vi "polhemus_only.vi"() -> ()   [LabVIEW 2017]
uses:
  <instrlib>/PDI/pdi.llb/PDI motion data.ctl
  <instrlib>/PDI/pdi.llb/PDI BINHDR.ctl
  <instrlib>/PDI/pdi.llb/PDI 6vec.ctl
  <instrlib>/PDI/pdi.llb/PDI counter.ctl
  <instrlib>/PDI/pdi.llb/PDI flag.ctl
  <instrlib>/PDI/pdi.llb/PDI DirCos cluster.ctl
  <instrlib>/PDI/pdi.llb/PDI quaternion.ctl
  <vilib>/Utility/file.llb/Write Delimited Spreadsheet (DBL).vi
panel:
  in  "file name":string
  in  "Path":path
  out "Continuing":bool
  in  "Stop Collect":bool
  out "motion data":T1 {"QT array"."Numeric 4" format="%_6g"; "QT array"."Numeric 3" format="%_6g"; "QT array"."Numeric 2" format="%_6g"; "QT array"."Numeric" format="%_6f"; "DC array"."Z"."z" format="%1_6f"; "DC array"."Z"."Y" format="%1_6f"; "DC array"."Z"."X" format="%1_6f"; "DC array"."Y"."z" format="%1_6f"; "DC array"."Y"."Y" format="%1_6f"; "DC array"."Y"."X" format="%1_6f"; "DC array"."X"."Z" format="%1_6f"; "DC array"."X"."Y" format="%1_6f"; "DC array"."X"."X" format="%1_6f"; "DL array" min=0 max=1 format="%.0g"; "ST array" min=0 max=1 format="%.0g"; "ES array" min=0 max=1 format="%.0g"; "TS array" format="%#.0g"; "FC array" format="%#.0g"; "XYZAER array"."R" format="%1_6f"; "XYZAER array"."E" format="%1_6f"; "XYZAER array"."A" format="%1_6f"; "XYZAER array"."Z" format="%1_6f"; "XYZAER array"."Y" format="%1_6f"; "XYZAER array"."X" format="%1_6f"; "BINHDR array"."Length" format="%04x"; "BINHDR array"."Reserved" format="%02x"; "BINHDR array"."Err" format="%02x"; "BINHDR array"."Cmd" format="%02x"; "BINHDR array"."Station" format="%02x"; "BINHDR array"."Preamble" format="%04x"}
  in  "Start Collect":bool
  in  "stop":bool
  out "error out":errorcluster {"code" format="%.0x"}
  out "Connected":bool
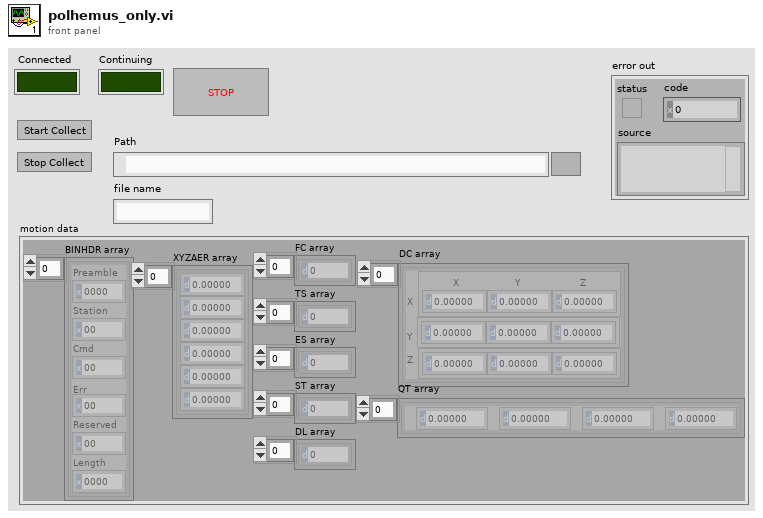
[diagram p1: front panel]
types:
  T1 = typedef "PDI motion data.ctl" = cluster{"BINHDR array":T2[], "XYZAER array":T3[], "FC array":T4[], "TS array":T4[], "ES array":T5[], "ST array":T5[], "DL array":T5[], "DC array":T6[], "QT array":T7[]}
  T2 = typedef "PDI BINHDR.ctl" = cluster{"Preamble":u16, "Station":u8, "Cmd":u8, "Err":u8, "Reserved":u8, "Length":u16}
  T3 = typedef "PDI 6vec.ctl" = cluster{"X":sgl, "Y":sgl, "Z":sgl, "A":sgl, "E":sgl, "R":sgl}
  T4 = typedef "PDI counter.ctl" = u32
  T5 = typedef "PDI flag.ctl" = i32
  T6 = typedef "PDI DirCos cluster.ctl" = cluster{"X":cluster{"X":sgl, "Y":sgl, "Z":sgl}, "Y":cluster{"X":sgl, "Y":sgl, "z":sgl}, "Z":cluster{"X":sgl, "Y":sgl, "z":sgl}}
  T7 = typedef "PDI quaternion.ctl" = cluster{"Numeric":sgl, "Numeric 2":sgl, "Numeric 3":sgl, "Numeric 4":sgl}
  T8 = enum16{"open", "open or create", "create or replace", "create", "open (read-only)"}
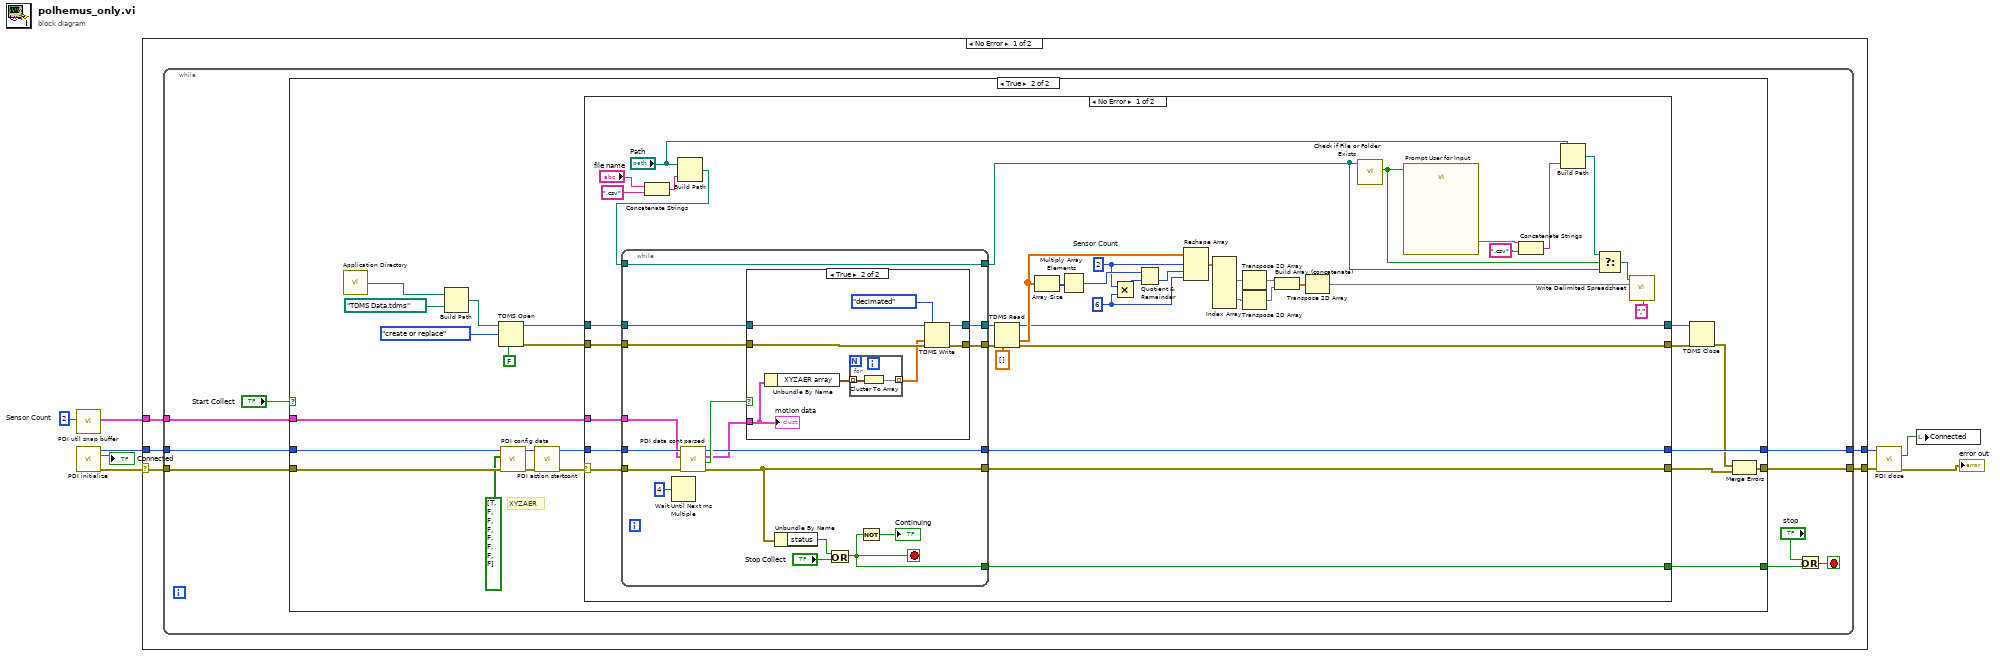
[diagram p0: block diagram]
diagram:
  w6 = 2  # Sensor Count
  n1 = call <instrlib>:"PDI util snap buffer.vi"("Sensor Count"=w6) -> ("snap buffer"=w7:T1)  [unwired: 8 in, 2 out]
  n2 = call <instrlib>:"PDI initialize.vi"() -> ("error out"=w4:errorcluster, "Connected"=→"Connected":bool, "pDev"=w8:u32)  [unwired: 5 in]
  n3 = case shown="No Error" w4 {
    selector: w4 -> [w11 w121]
    tunnel: [w14 w121] -> w3
    tunnel: [w13 w122] -> w5
    tunnel: w8 -> [w10 w122]
    tunnel: w7 -> [w12 _]
    frame No Error {
      n4 = while {
        tunnel: [w21] -> w14
        tunnel: [w20] -> w13
        tunnel: w12 -> [w19]
        tunnel: w11 -> [w18]
        tunnel: w10 -> [w17]
        stop <- w16 stop-if-true
        n5 = case shown="True" "Start Collect" {
          tunnel: [w24 w38] -> w21
          tunnel: [w25 w47] -> w20
          tunnel: w19 -> [_ w46]
          tunnel: w18 -> [w24 w32]
          tunnel: w17 -> [w25 w30]
          tunnel: [_ w27] -> w15
          frame False {
          }
          frame True {
            # "XYZAER"
            n6 = call <vilib>:"Application Directory.vi"() -> ("Application Directory"=w26:path)
            n7 = Build Path(base path=w26, name or relative path=path "TDMS Data.tdms" ("file path")) -> (appended path=w41:path)
            n8 = TDMS Open(6:FALSE ("disable buffering? (T)"), 10:T8."create or replace" ("operation"), 11:w41) -> (0:w44:errorcluster, 3:w45:refnum<k34>)  [unwired: 4 in]
            n9 = call <instrlib>:"PDI config data.vi"("error in (no error)"=w32, "Frame Data Select\nXYZAER    FC           TS           ES          ST           DL          DC          QT"=bool[] [TRUE, FALSE, FALSE, FALSE, FALSE, FALSE, FALSE, FALSE] ("Frame Data Select\nXYZAER    FC           TS           ES          ST           DL          DC          QT"), "pDev"=w30) -> ("error out"=w33:errorcluster, "dup pDev"=w34:u32)  [unwired: 5 in, 2 out]
            n10 = call <instrlib>:"PDI action startcont.vi"("error in (no error)"=w33, "pDev"=w34) -> ("error out"=w29:errorcluster, "dup pDev"=w28:u32)  [unwired: 7 in, 1 out]
            n11 = case shown="No Error" w29 {
              selector: w29 -> [w87 w120]
              tunnel: [w83 w120] -> w39
              tunnel: w28 -> [w86 w119]
              tunnel: [w84 w119] -> w47
              tunnel: w46 -> [w85 _]
              tunnel: w45 -> [w82 w118]
              tunnel: [w61 w118] -> w36
              tunnel: [w62 w117] -> w35
              tunnel: w44 -> [w81 w117]
              tunnel: [w60 _] -> w27
              frame No Error {
                w75 = 2  # Sensor Count
                w74 = 6 ("dimension size")
                n12 = Concatenate Strings("file name", ".csv" ("string")) -> (w58:string)
                n13 = Build Path(base path="Path", name or relative path=w58) -> (appended path=w49:path)
                n14 = while {
                  tunnel: w87 -> [w103]
                  tunnel: w86 -> [w104]
                  tunnel: w85 -> [w101]
                  tunnel: [w100] -> w84
                  tunnel: [w97] -> w83
                  tunnel: w82 -> [w96]
                  tunnel: [w95] -> w65
                  tunnel: [w94] -> w63
                  tunnel: w81 -> [w93]
                  tunnel: [w89] -> w60
                  tunnel: w49 -> [w88]
                  tunnel: [w88] -> w48
                  stop <- w89 stop-if-true
                  n15 = Wait Until Next ms Multiple(millisecond multiple=u32 4) -> ()  [unwired: 1 out]
                  n16 = call <instrlib>:"PDI data cont parsed.vi"("error in (no error)"=w103, "motion data IN"=w101, "pDev"=w104) -> ("error out"=w97:errorcluster, "DataReady"=w102:bool, "motion data OUT"=w92:T1, "dup pDev"=w100:u32)  [unwired: 4 in, 1 out]
                  n17 = case shown="True" w102 {
                    tunnel: w92 -> [_ w110]
                    tunnel: w96 -> [w106 w114]
                    tunnel: [w106 w113] -> w95
                    tunnel: [w105 w112] -> w94
                    tunnel: w93 -> [w105 w111]
                    frame False {
                    }
                    frame True {
                      n18 = Unbundle By Name(w110) -> ("XYZAER array"=w109:T3[])
                      n19 = for {
                        tunnel: w109 -> [w116] mode=indexing
                        tunnel: [w115] -> w108 mode=indexing
                        n20 = Cluster To Array(cluster=w116) -> (array=w115:sgl[])
                      }
                      n21 = TDMS Write(0:w114, 1:enum16{"decimated", "interleaved"}."decimated" ("data layout (0:decimated)"), 9:w108, 11:w111) -> (4:w113:refnum<k34>, 15:w112:errorcluster)  [unwired: 2 in, 2 out]
                      "motion data" <- w110
                    }
                  }
                  n22 = Unbundle By Name(w97) -> ("status"=w98:bool)
                  n23 = Or(x=w98, y="Stop Collect") -> (x .or. y?=w89:bool)
                  n24 = Not(x=w89) -> (.not. x?=→"Continuing":bool)
                }
                n25 = TDMS Read(0:w65, 11:w63, 12:sgl[][] [] ("6VEC")) -> (4:w61:refnum<k34>, 10:w80:sgl[][], 15:w62:errorcluster)  [unwired: 5 in, 3 out]
                n26 = Array Size(array=w80) -> (size(s)=w79:i32[])
                n27 = Multiply Array Elements(1:w79) -> (0:w78:i32)
                n28 = Multiply(x=w75, y=w74) -> (x*y=w76:i32)
                n29 = Quotient & Remainder(x=w78, y=w76) -> (floor(x/y)=w77:i32)  [unwired: 1 out]
                n30 = Reshape Array(w80, w75, w77, w74) -> (w73:sgl[][][])
                n31 = Index Array(array=w73) -> (element #1=w72:sgl[][], element #2=w71:sgl[][])  [unwired: 6 in]
                n32 = Transpose 2D Array(2D array=w72) -> (transposed array=w69:sgl[][])
                n33 = Transpose 2D Array(2D array=w71) -> (transposed array=w68:sgl[][])
                n34 = Build Array (concatenate)(w69, w68) -> (w70:sgl[][])
                n35 = Transpose 2D Array(2D array=w70) -> (transposed array=w67:sgl[][])
                n36 = call <vilib>:"Check if File or Folder Exists.vi"("path"=w48) -> ("file or folder exists?"=w52:bool)  [unwired: 8 in, 2 out]
                n37 = call "Prompt User for Input"("Enable"=w52) -> ("File name"=w50:string)  [unwired: 16 in, 2 out]
                n38 = Concatenate Strings(w50, ".csv" ("string")) -> (w55:string)
                n39 = Build Path(base path="Path", name or relative path=w55) -> (appended path=w53:path)
                n40 = Select(t=w53, s=w52, f=w48) -> (s? t:f=w56:path)
                n41 = call-poly <vilib>:"Write Delimited Spreadsheet.vi"("file path (dialog if empty)"=w56, "2D data"=w67, "delimiter (\\t)"="," ("delimiter (\\t)")) -> ()  [unwired: 11 in, 2 out]
              }
              frame Error {
              }
            }
            n42 = TDMS Close(8:w35, 11:w36) -> (0:w37:errorcluster)  [unwired: 1 out]
            n43 = Merge Errors(w37, w39) -> (w38:errorcluster)
          }
        }
        n44 = Or(x="stop", y=w15) -> (x .or. y?=w16:bool)
      }
    }
    frame Error {
    }
  }
  n45 = call <instrlib>:"PDI close.vi"("error in (no error)"=w3, "pDev"=w5) -> ("error out"=→"error out":errorcluster, "connected"=w1:bool)  [unwired: 8 in]
  n46 = local write "Connected"(w1) -> ()
